vi "SMU_IV single.vi"() -> ()   [LabVIEW 2022 SP3]
uses:
  <vilib>/Analysis/1siggen.llb/Ramp Pattern by Delta.vi
  Agilent U2722/Public/Configure/Configure Channel (Current).vi
  Agilent U2722/Public/Configure/Configure Channel (Voltage).vi
  Agilent U2722/Public/Data/Read Output (Single).vi
  <vilib>/Utility/file.llb/Write Delimited Spreadsheet (DBL).vi
  Agilent U2722/Agilent U2722.lvlib
  <vilib>/Analysis/NI_AALBase.lvlib
panel:
  in  "Tab Control":enum32{"Device Setup"}(tab)
  in  "Voltage Range 2":u16(ring) items=["2 Volts", "20 Volts"]
  in  "Current Range 2":u16(ring)=4 items=["1 uA", "10 uA", "100 uA", "1 mA", "10 mA", "120 mA"]
  in  "Current Limit  2":dbl=0.005 format="%#_2p"
  in  "Voltage Range":u16(ring) items=["2 Volts", "20 Volts"]
  in  "Starting Voltage (V)":dbl
  in  "Stopping Voltage (V)":dbl=1.0
  in  "Voltage Interval  (DV)":dbl format="%#_2g"
  in  "Current Range":u16(ring)=4 items=["1 uA", "10 uA", "100 uA", "1 mA", "10 mA", "120 mA"]
  in  "VISA resource name":refnum<visa-resource-name>
  in  "Drain - Source Channel":u16(ring)=1 items=["Channel 1"=1, "Channel 2"=2, "Channel 3"=3]
  in  "PLC":i32
  in  "Current Limit":dbl=0.005 format="%#_2p"
  in  "Interval Time (s)":dbl=1.0 caption="Delay Time (s)"
  in  "Starting Voltage (V) 2":dbl
  in  "Stopping Voltage (V) 2":dbl=1.0
  in  "Voltage Interval 2 (DV)":dbl format="%#_2g"
  in  "Gate - Source Channel":u16(ring)=2 items=["Channel 1"=1, "Channel 2"=2, "Channel 3"=3]
  in  "output file path":path
  out "XY Graph":cluster{"Y":dbl[], "Y":dbl[]}[](graph)
  out "XY Graph 2":cluster{"Y":dbl[], "Y":dbl[]}[](graph)
  # "Drain Source Voltage Setting"
  # "Gate Source Voltage Setting"
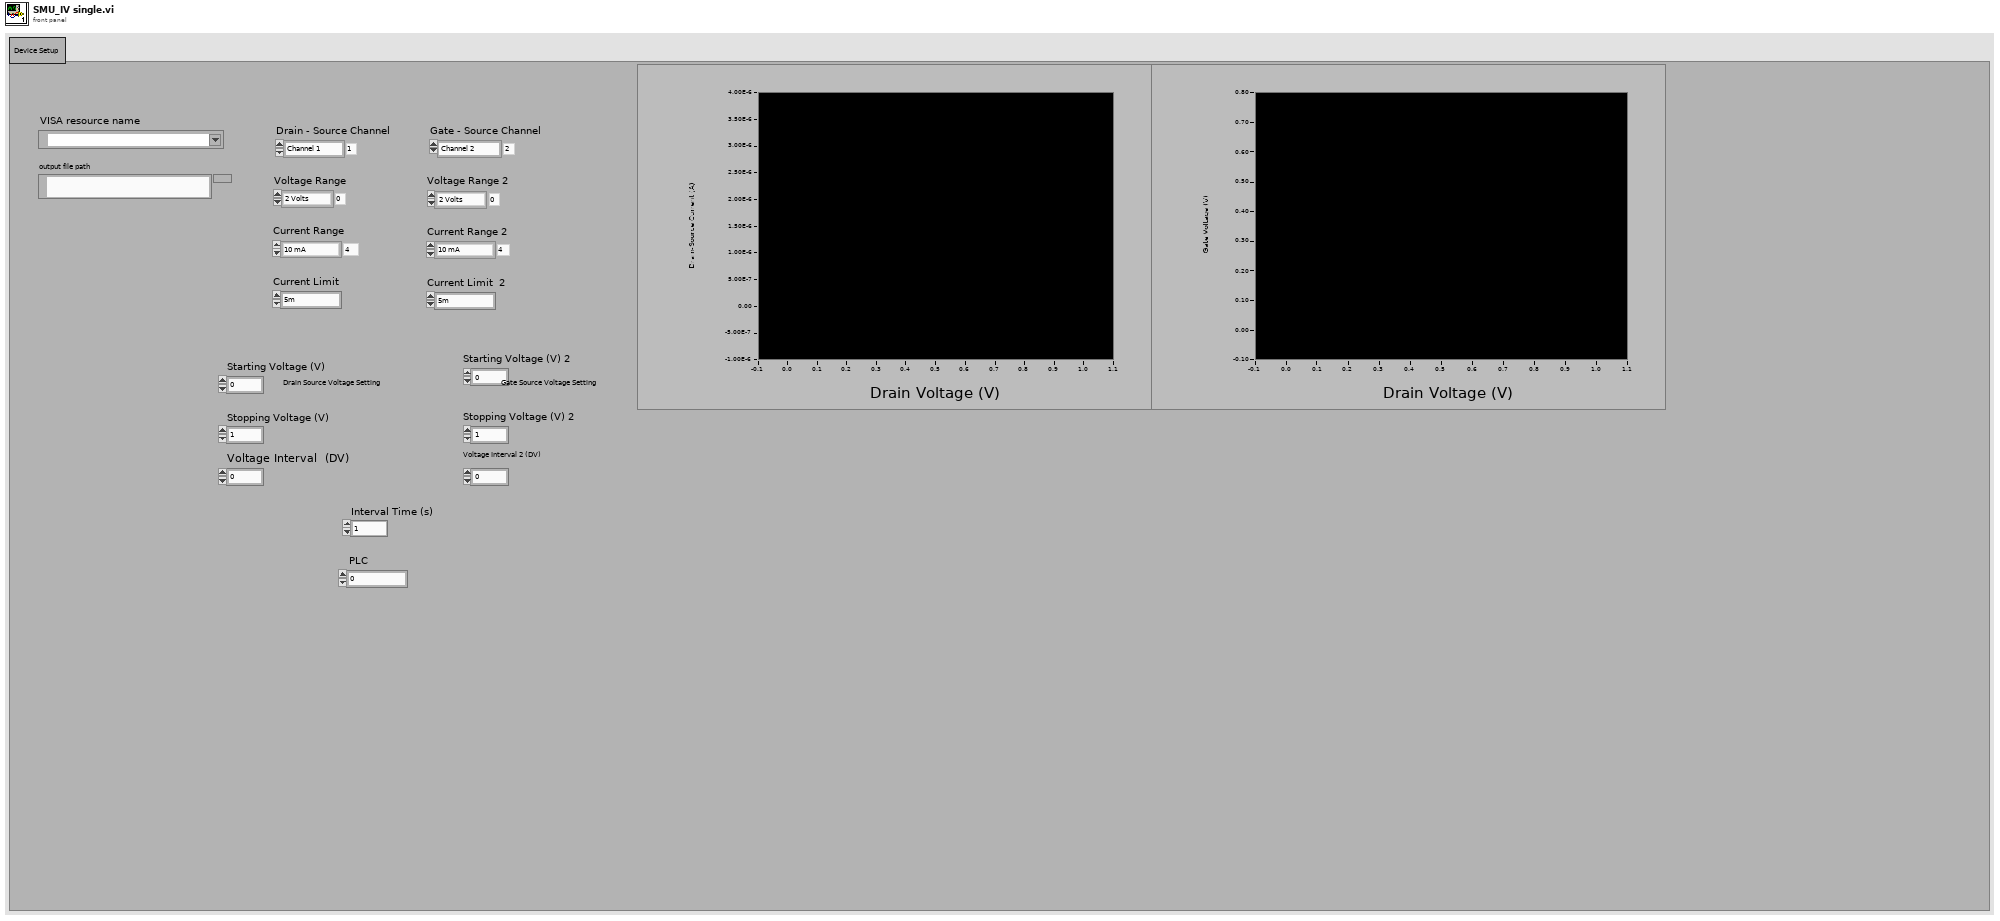
[diagram p1: front panel]
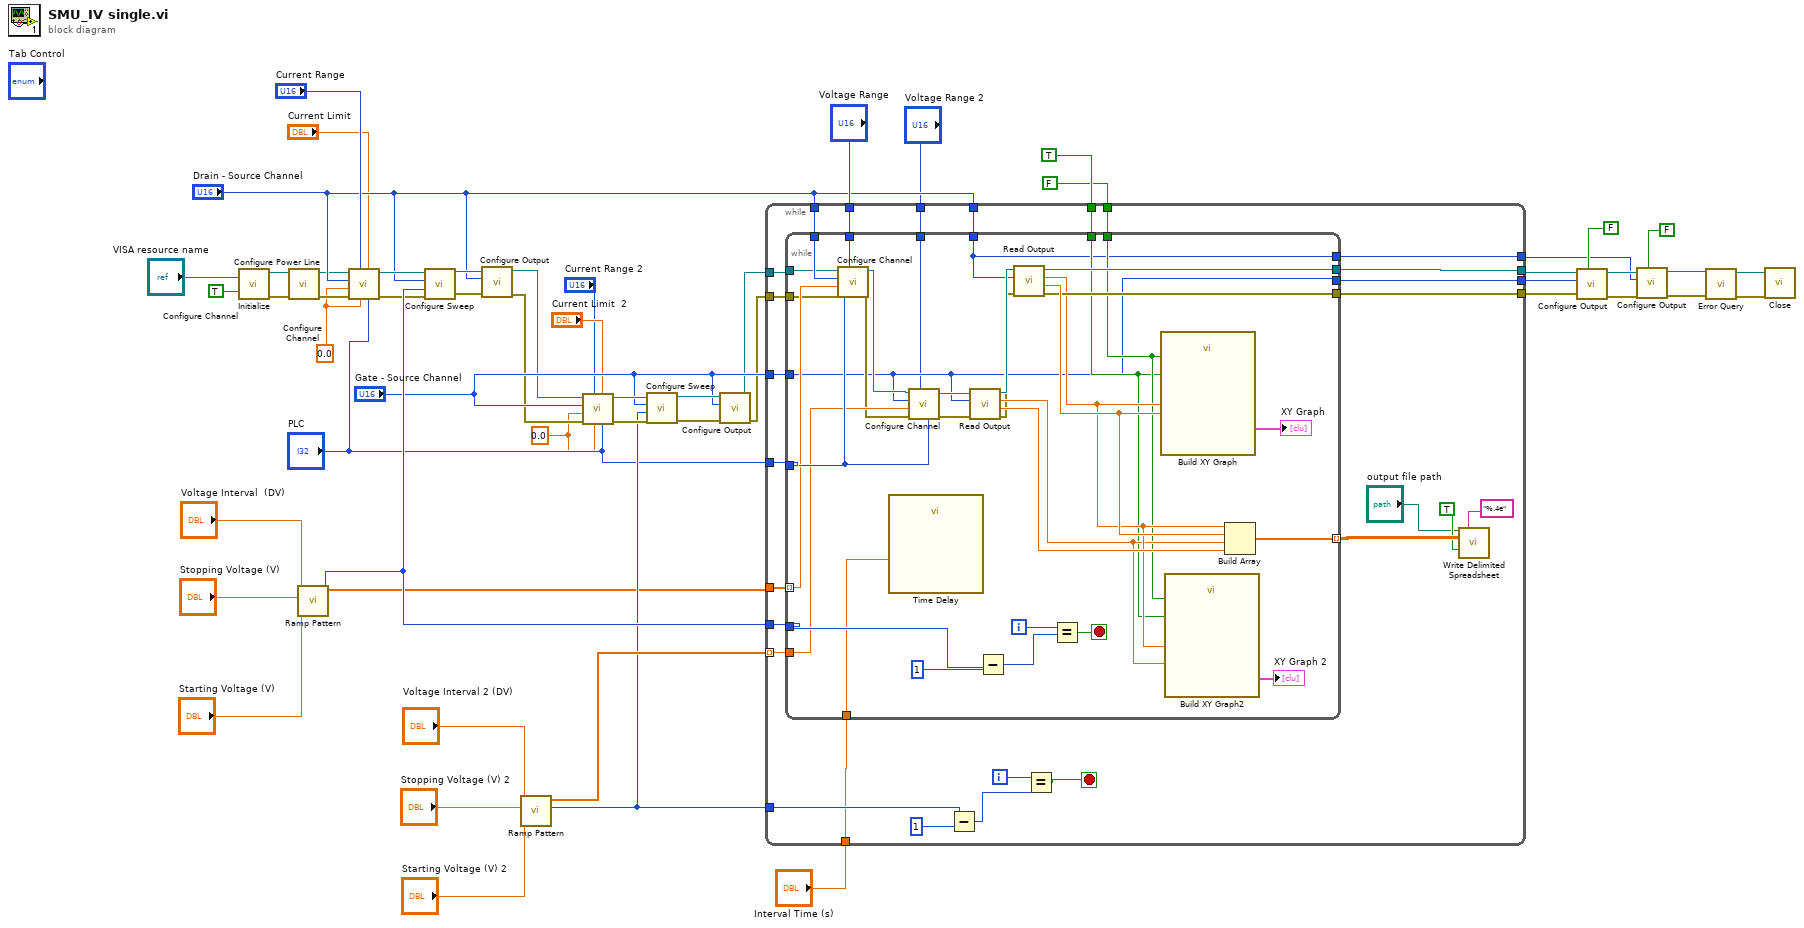
[diagram p0: block diagram]
diagram:
  w3 = 0.0
  w2 = 0.0
  n1 = call "Initialize.vi"("ID Query (True)"=TRUE, "VISA resource name"="VISA resource name") -> ("error out"=w49:errorcluster, "VISA resource name out"=w48:refnum<visa-resource-name>)  [unwired: 8 in]
  n2 = call "Configure Power Line.vi"("error in (no error)"=w49, "VISA resource name"=w48) -> ("error out"=w32:errorcluster, "VISA resource name out"=w19:refnum<visa-resource-name>)  [unwired: 8 in]
  n3 = call-poly <vilib>:"Ramp Pattern.vi"("start"="Starting Voltage (V)", "end"="Stopping Voltage (V)", "delta"="Voltage Interval  (DV)") -> ("samples"=w39:i32, "Ramp Pattern"=w22:dbl[])  [unwired: 6 in, 1 out]
  n4 = call-poly "Configure Channel.vi"("Power Line Cycles (0)"="PLC", "Current Limit (1.0 uA)"="Current Limit", "Triggered Level (1.0 mA)"=w2, "Current Range (0: 1 uA)"="Current Range", "error in (no error)"=w32, "Output Level (1.0 mA)"=w2, "Channel (1: Channel 1)"="Drain - Source Channel", "VISA resource name"=w19) -> ("error out"=w36:errorcluster, "VISA resource name out"=w37:refnum<visa-resource-name>)  [unwired: 2 in]
  n5 = call "Configure Sweep.vi"("error in (no error)"=w36, "Sweep Points (1)"=w39, "Channel (1: Channel 1)"="Drain - Source Channel", "VISA resource name"=w37) -> ("error out"=w40:errorcluster, "VISA resource name out"=w41:refnum<visa-resource-name>)  [unwired: 6 in]
  n6 = call "Configure Output.vi"("error in (no error)"=w40, "Channel (1: Channel 1)"="Drain - Source Channel", "VISA resource name"=w41) -> ("error out"=w17:errorcluster, "VISA resource name out"=w18:refnum<visa-resource-name>)  [unwired: 7 in]
  n7 = call-poly <vilib>:"Ramp Pattern.vi"("start"="Starting Voltage (V) 2", "end"="Stopping Voltage (V) 2", "delta"="Voltage Interval 2 (DV)") -> ("samples"=w25:i32, "Ramp Pattern"=w26:dbl[])  [unwired: 6 in, 1 out]
  n8 = call-poly "Configure Channel.vi"("Power Line Cycles (0)"="PLC", "Current Limit (1.0 uA)"="Current Limit  2", "Triggered Level (1.0 mA)"=w3, "Current Range (0: 1 uA)"="Current Range 2", "error in (no error)"=w17, "Output Level (1.0 mA)"=w3, "Channel (1: Channel 1)"="Gate - Source Channel", "VISA resource name"=w18) -> ("error out"=w31:errorcluster, "VISA resource name out"=w30:refnum<visa-resource-name>)  [unwired: 2 in]
  n9 = call "Configure Sweep.vi"("error in (no error)"=w31, "Sweep Points (1)"=w25, "Channel (1: Channel 1)"="Gate - Source Channel", "VISA resource name"=w30) -> ("error out"=w28:errorcluster, "VISA resource name out"=w29:refnum<visa-resource-name>)  [unwired: 6 in]
  n10 = call "Configure Output.vi"("error in (no error)"=w28, "Channel (1: Channel 1)"="Gate - Source Channel", "VISA resource name"=w29) -> ("error out"=w16:errorcluster, "VISA resource name out"=w15:refnum<visa-resource-name>)  [unwired: 7 in]
  n11 = while {
    tunnel: TRUE -> [w81]
    tunnel: FALSE -> [w80]
    tunnel: "PLC" -> [w79]
    tunnel: "Interval Time (s)" -> [w64]
    tunnel: w39 -> [w78]
    tunnel: "Voltage Range" -> [w77]
    tunnel: "Gate - Source Channel" -> [w76]
    tunnel: w26 -> [w75] mode=indexing
    tunnel: w25 -> [w71]
    tunnel: [w69] -> w24
    tunnel: [w68] -> w23
    tunnel: w22 -> [w67]
    tunnel: "Drain - Source Channel" -> [w66]
    tunnel: "Drain - Source Channel" -> [w65]
    tunnel: w16 -> [w56]
    tunnel: w15 -> [w63]
    tunnel: [w58] -> w9
    tunnel: [w57] -> w8
    tunnel: "Voltage Range 2" -> [w55]
    i -> [w73]
    stop <- w72 stop-if-true
    n12 = while {
      tunnel: w78 -> [w111]
      tunnel: w64 -> [w110]
      tunnel: w79 -> [w106]
      tunnel: w81 -> [w87]
      tunnel: w80 -> [w88]
      tunnel: [w95] -> w69
      tunnel: [w108] -> w68
      tunnel: w76 -> [w86]
      tunnel: w77 -> [w83]
      tunnel: w75 -> [w105]
      tunnel: [w98] -> w61 mode=indexing
      tunnel: w67 -> [w97] mode=indexing
      tunnel: w66 -> [w96]
      tunnel: w65 -> [w85]
      tunnel: w63 -> [w92]
      tunnel: [w86] -> w58
      tunnel: [w85] -> w57
      tunnel: w56 -> [w84]
      tunnel: w55 -> [w82]
      i -> [w107]
      stop <- w109 stop-if-true
      n13 = call-poly "Configure Channel.vi"("Power Line Cycles (0)"=w106, "Voltage Range (0: 2 Volts)"=w83, "error in (no error)"=w84, "Output Level (1.0 V)"=w97, "Channel (1: Channel 1)"=w96, "VISA resource name"=w92) -> ("error out"=w90:errorcluster, "VISA resource name out"=w91:refnum<visa-resource-name>)  [unwired: 4 in]
      n14 = call "Time Delay"("Delay Time (s)"=w110) -> ()  [unwired: 10 in, 1 out]
      n15 = call-poly "Configure Channel.vi"("Power Line Cycles (0)"=w106, "Voltage Range (0: 2 Volts)"=w82, "error in (no error)"=w90, "Output Level (1.0 V)"=w105, "Channel (1: Channel 1)"=w86, "VISA resource name"=w91) -> ("error out"=w103:errorcluster, "VISA resource name out"=w104:refnum<visa-resource-name>)  [unwired: 4 in]
      n16 = call-poly "Read Output.vi"("error in (no error)"=w103, "Channel (1: Channel 1)"=w86, "VISA resource name"=w104) -> ("error out"=w89:errorcluster, "Actual Current Level (A)"=w102:dbl, "Actual Voltage Level (V)"=w94:dbl, "VISA resource name out"=w93:refnum<visa-resource-name>)  [unwired: 5 in]
      n17 = Subtract(x=w111, y=1 ("x")) -> (x-y=w113:i32)
      n18 = call-poly "Read Output.vi"("error in (no error)"=w89, "Channel (1: Channel 1)"=w85, "VISA resource name"=w93) -> ("error out"=w108:errorcluster, "Actual Current Level (A)"=w112:dbl, "Actual Voltage Level (V)"=w100:dbl, "VISA resource name out"=w95:refnum<visa-resource-name>)  [unwired: 5 in]
      n19 = Equal?(x=w107, y=w113) -> (x = y?=w109:bool)
      n20 = call "Build XY Graph"("Enable"=w87, "Reset"=w88, "Y Input"=w112, "X Input"=w100) -> ("XY Graph"=→"XY Graph":cluster{"X":dbl[], "Y":dbl[]}[])  [unwired: 6 in, 1 out]
      n21 = call "Build XY Graph2"("Enable"=w87, "Reset"=w88, "Y Input"=w94, "X Input"=w100) -> ("XY Graph"=→"XY Graph 2":cluster{"X":dbl[], "Y":dbl[]}[])  [unwired: 6 in, 1 out]
      n22 = Build Array(w100, w112, w94, w102) -> (w98:dbl[])
    }
    n23 = Subtract(x=w71, y=1 ("x")) -> (x-y=w70:i32)
    n24 = Equal?(x=w73, y=w70) -> (x = y?=w72:bool)
    n25 = call-poly <vilib>:"Write Delimited Spreadsheet.vi"("file path (dialog if empty)"="output file path", "format (%.3f)"="%.4e", "2D data"=w61, "append to file? (new file:F)"=TRUE) -> ()  [unwired: 10 in, 2 out]
  }
  n26 = call "Configure Output.vi"("Enable Output (T: Enable)"=FALSE, "error in (no error)"=w23, "Channel (1: Channel 1)"=w9, "VISA resource name"=w24) -> ("error out"=w12:errorcluster, "VISA resource name out"=w14:refnum<visa-resource-name>)  [unwired: 6 in]
  n27 = call "Configure Output.vi"("Enable Output (T: Enable)"=FALSE, "error in (no error)"=w12, "Channel (1: Channel 1)"=w8, "VISA resource name"=w14) -> ("error out"=w11:errorcluster, "VISA resource name out"=w13:refnum<visa-resource-name>)  [unwired: 6 in]
  n28 = call "Error Query.vi"("error in (no error)"=w11, "VISA resource name"=w13) -> ("error out"=w43:errorcluster, "VISA resource name out"=w42:refnum<visa-resource-name>)  [unwired: 6 in, 2 out]
  n29 = call "Close.vi"("error in (no error)"=w43, "VISA resource name"=w42) -> ()  [unwired: 9 in, 1 out]
